vi "Write Prefix.vi"(8 "error in":errorcluster, 10 "Replacement":string, 11 "Regex Scrubber in":refnum<class "Regex Scrubber Count Unique.lvclass">) -> (0 "error out":errorcluster, 3 "Regex Scrubber out":refnum<class "Regex Scrubber Count Unique.lvclass">)   [LabVIEW 2020, in "Approval Tests.lvlib" / "Regex Scrubber Count Unique.lvclass"]
uses:
  Regex Scrubber Count Unique.lvclass
  Regex Scrubber Count Unique.lvclass/Regex Scrubber Count Unique.ctl
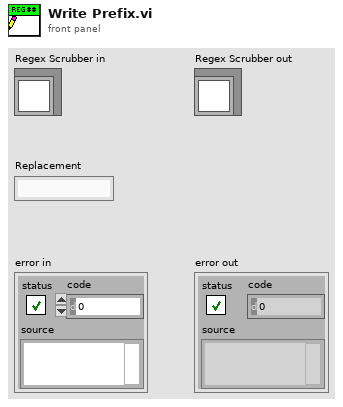
[diagram p1: front panel]
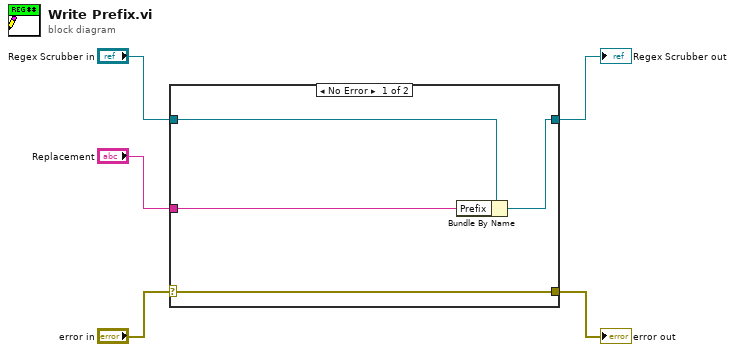
[diagram p0: block diagram]
diagram:
  n1 = case shown="No Error" "error in" {
    selector: "error in" -> [w9 w11]
    tunnel: [w9 w11] -> w4
    tunnel: [w7 w10] -> w2
    tunnel: "Regex Scrubber in" -> [w8 w10]
    tunnel: "Replacement" -> [w6 _]
    frame No Error {
      n2 = Bundle By Name(cluster=w8, "Prefix"=w6) -> (w7:refnum<class "Regex Scrubber Count Unique.lvclass">)
    }
    frame Error {
    }
  }
  "error out" <- w4
  "Regex Scrubber out" <- w2
